vi "_getViBookmarksInfo.vi"(8 "error in (no error)":errorcluster, 11 "VI in":refnum<vi>) -> (0 "error out":errorcluster, 2 "Bookmarks":string[][](array[string]), 3 "VI out":refnum<vi>)   [LabVIEW 2017]
doc: "Returns the bookmark information for the specified VI reference."
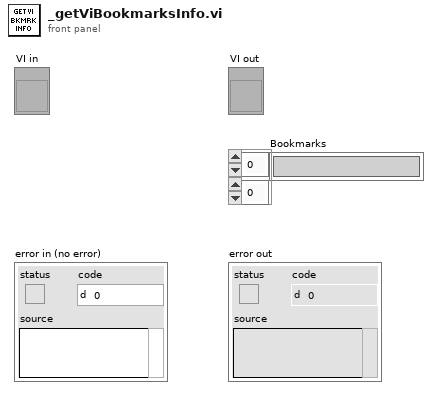
[diagram p1: front panel]
types:
  T1 = typedef "LVBookmarkInfoTypeDef.ctl" = cluster{"Bookmark Reference":u32, "Bookmark Tag":string, "Label Text":string}[]
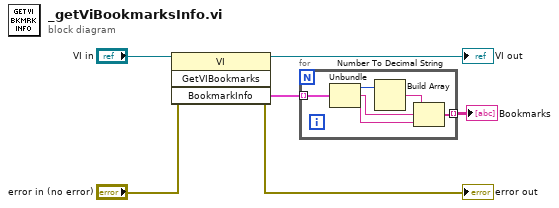
[diagram p0: block diagram]
diagram:
  n1 = invoke class="VI" method="GetVIBookmarks"(reference="VI in", error in="error in (no error)") -> (reference out=→"VI out":refnum<vi>, error out=→"error out":errorcluster, "BookmarkInfo"=w2:T1)  [unwired: 2 in, 1 out]
  n2 = for {
    tunnel: w2 -> [w12] mode=indexing
    tunnel: [w7] -> w1 mode=indexing
    n3 = Unbundle(w12) -> ("Bookmark Reference"=w11:u32, "Bookmark Tag"=w9:string, "Label Text"=w8:string)
    n4 = Number To Decimal String(number=w11) -> (decimal integer string=w10:string)  [unwired: 1 in]
    n5 = Build Array(w10, w9, w8) -> (w7:string[])
  }
  "Bookmarks" <- w1
